vi "PassPlay_v2_Init.vi"(0 "object in":refnum<class "PassPlay_v2.lvclass">, 5 "error in (no error)":errorcluster) -> (14 "object out":refnum<class "PassPlay_v2.lvclass">, 19 "error out":errorcluster)   [LabVIEW 2023, in "PassPlay_v2.lvclass"]
uses:
  PassPlay_v2.lvclass
  C:/Users/ebert/Documents/codes/SSL/repo/SSL_AI/NewSTP/NewPlays/Play_v2_class/Play_v2.lvclass
  NewRoles/PassReceiver_v2_class/PassReceiver_v2.lvclass
  C:/Users/ebert/Documents/codes/SSL/repo/SSL_AI/NewSTP/NewRoles/Role_v2_class/Role_v2.lvclass
  Play_v2_class/Play_v2.lvclass
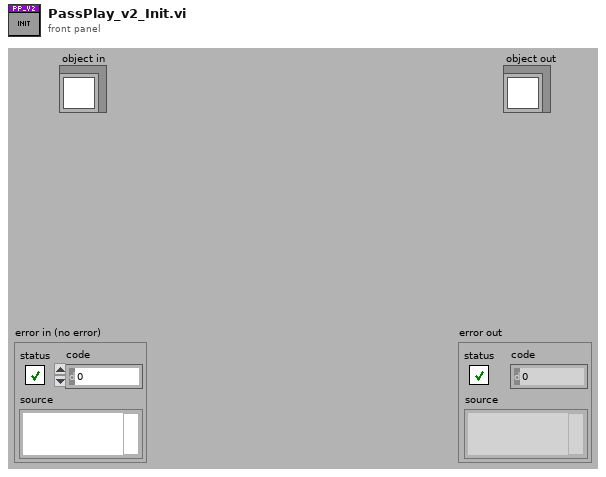
[diagram p1: front panel]
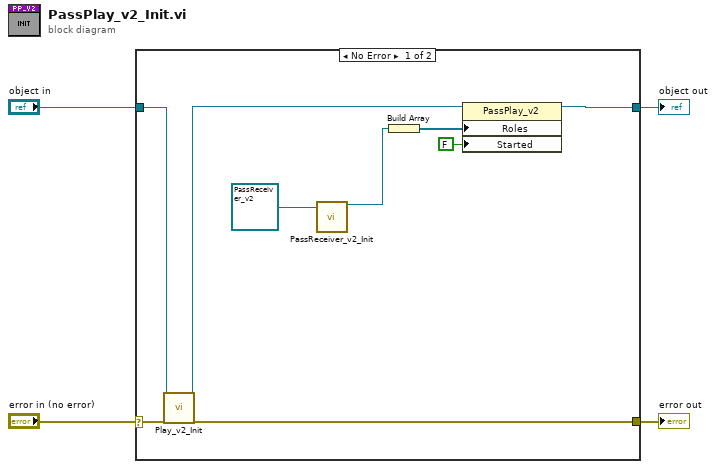
[diagram p0: block diagram]
diagram:
  n1 = case shown="No Error" "error in (no error)" {
    selector: "error in (no error)" -> [w13 w14]
    tunnel: [w9 w15] -> w4
    tunnel: "object in" -> [w11 w15]
    tunnel: [w12 w14] -> w1
    frame No Error {
      n2 = call "Play_v2_Init.vi"("object in"=w11, "error in (no error)"=w13) -> ("object out"=w10:refnum<class "PassPlay_v2.lvclass">, "error out"=w12:errorcluster)  [unwired: 16 in]
      n3 = call "PassReceiver_v2_Init.vi"("object in"=refnum<class "PassReceiver_v2.lvclass"> refnum ("PassReceiver_v2")) -> ("object out"=w5:refnum<class "PassReceiver_v2.lvclass">)  [unwired: 17 in, 1 out]
      n4 = Build Array(w5) -> (w7:refnum<class "PassReceiver_v2.lvclass">[])
      n5 = property class="PassPlay_v2"(reference=w10, "Roles"=w7, "Started"=FALSE) -> (reference out=w9:refnum<class "PassPlay_v2.lvclass">)  [unwired: 1 in, 1 out]
    }
    frame Error {
    }
  }
  "object out" <- w4
  "error out" <- w1
